vi "Get logging.vi"(8 "error in (no error)":errorcluster, 11 "ConfocalStage in":refnum<class "ConfocalStage.lvclass">) -> (0 "error out":errorcluster, 2 "logging?":bool, 3 "ConfocalStage out":refnum<class "ConfocalStage.lvclass">)   [LabVIEW 2012, in "ConfocalStage.lvclass"]
uses:
  ConfocalStage.lvclass
  ConfocalStage.lvclass/ConfocalStage.ctl
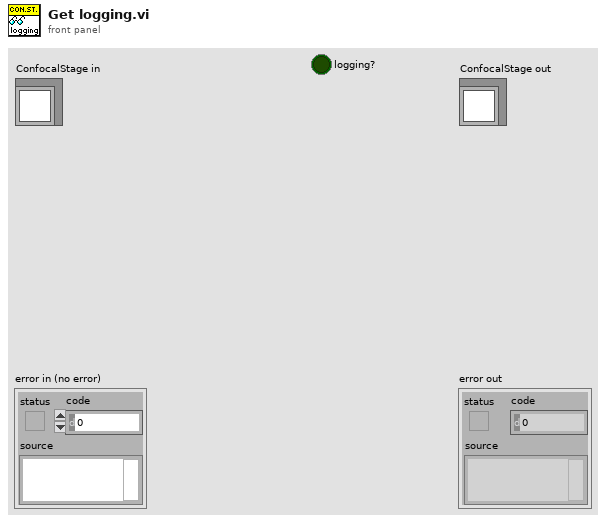
[diagram p1: front panel]
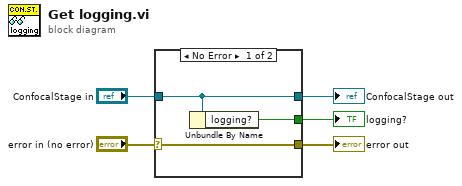
[diagram p0: block diagram]
diagram:
  n1 = case shown="No Error" "error in (no error)" {
    selector: "error in (no error)" -> [w8 w10]
    tunnel: [w8 w10] -> w4
    tunnel: [w7 w9] -> w2
    tunnel: "ConfocalStage in" -> [w7 w9]
    tunnel: [w6 _] -> w1
    frame No Error {
      n2 = Unbundle By Name(w7) -> ("logging?"=w6:bool)
    }
    frame Error {
    }
  }
  "error out" <- w4
  "ConfocalStage out" <- w2
  "logging?" <- w1
